vi "PicoScope6000aGetTriggerInfo.vi"(0 "handle in":i16, 5 "Segment Range":T1={"fromSegmentIndex"=0, "toSegmentIndex"=9} {"toSegmentIndex" format="%.4p"; "fromSegmentIndex" format="%.4p"}, 9 "Sample Rate":dbl, 11 "error in":errorcluster) -> (4 "handle out":i16, 6 "Trigger Info":T2(array[cluster]), 10 "Trigger Offsets":cluster{"Samples":u64, "Time (seconds)":dbl}[](array[cluster]) {"Time (seconds)" format="%#_5p"}, 15 "error out":errorcluster)   [LabVIEW 2010]
doc: "This VI gets a set of blocks captured using rapid block mode. It outputs two-dimensional arrays for each channel that contain data from all the requested captures."
uses:
  ps6000a.dll
  shared/Segment Range.ctl
panel:
  out "Number of Captures":u64=1
  out "fromSegmentIndex":u64
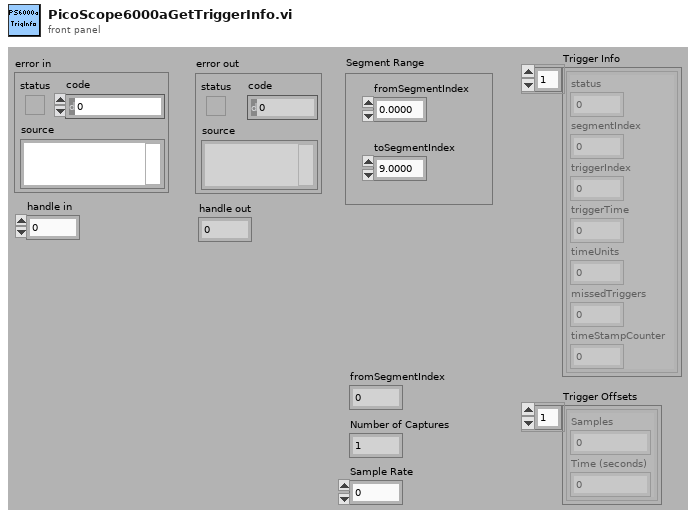
[diagram p1: front panel]
types:
  T1 = typedef "Segment Range.ctl" = cluster{"fromSegmentIndex":u64, "toSegmentIndex":u64}
  T2 = cluster{"status":u32, "segmentIndex":u64, "triggerIndex":u64, "triggerTime":dbl, "timeUnits":u32, "missedTriggers":u64, "timeStampCounter":u64}[]
  T3 = cluster{"status":u32, "segmentIndex":u64, "triggerIndex":u64, "triggerTime":dbl, "timeUnits":u32, "missedTriggers":u64, "timeStampCounter":u64}
  T4 = cluster{"status":bool, "code":u32, "source":string}
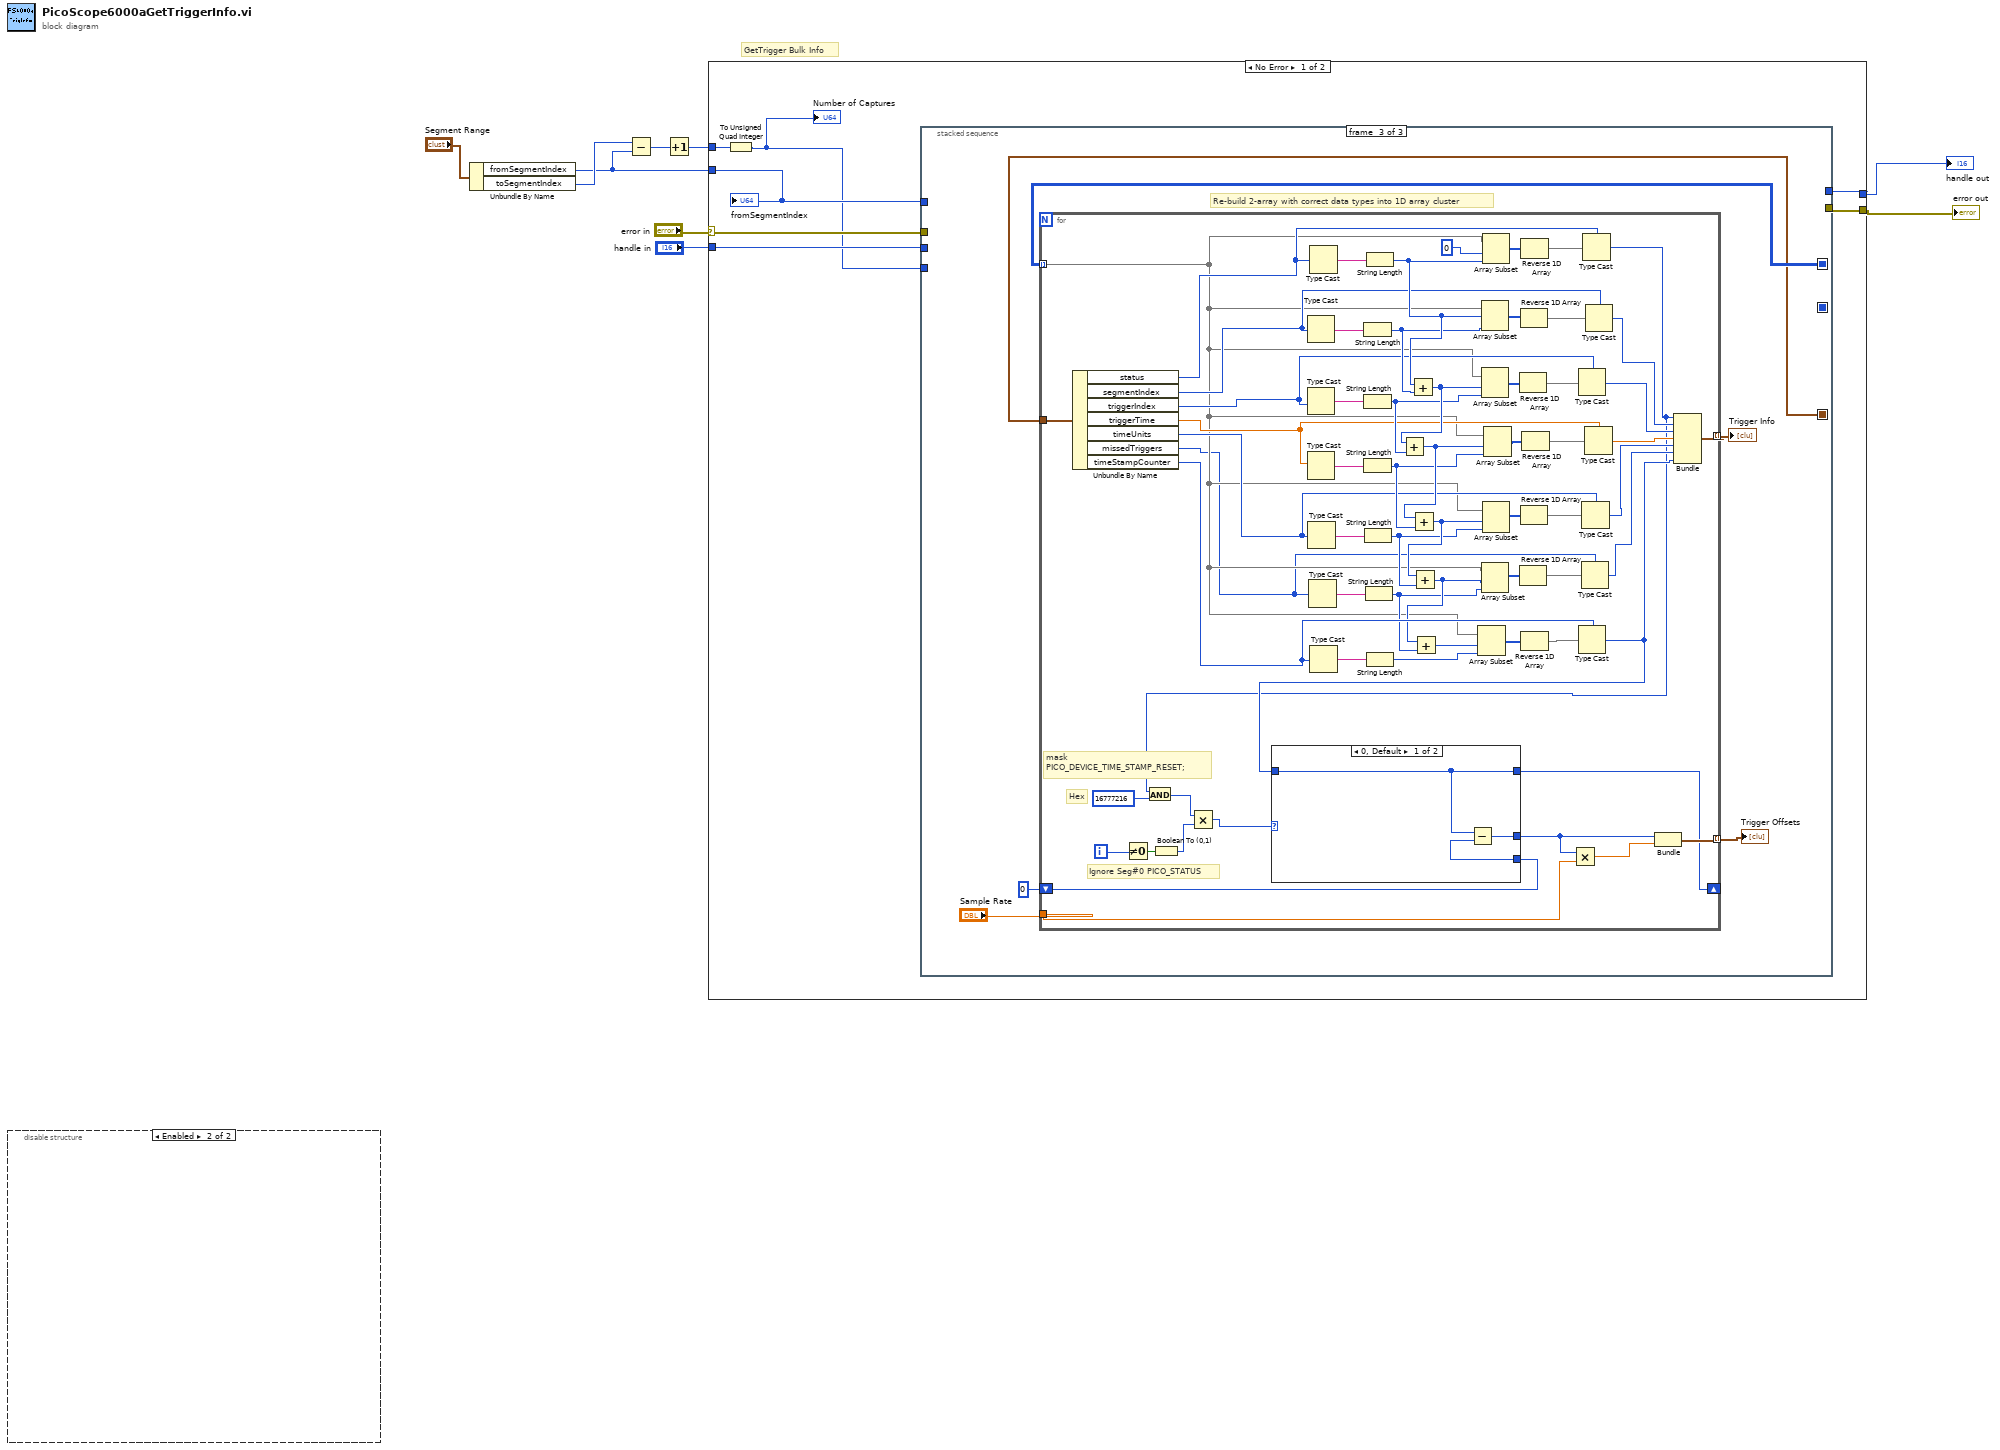
[diagram p0: block diagram]
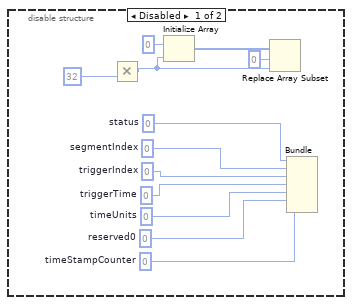
[diagram p2: hidden frame]
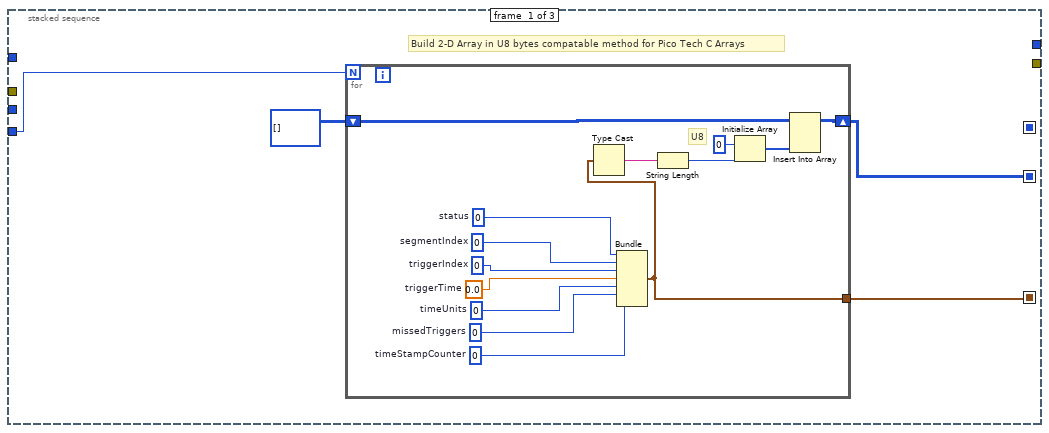
[diagram p3: hidden frame]
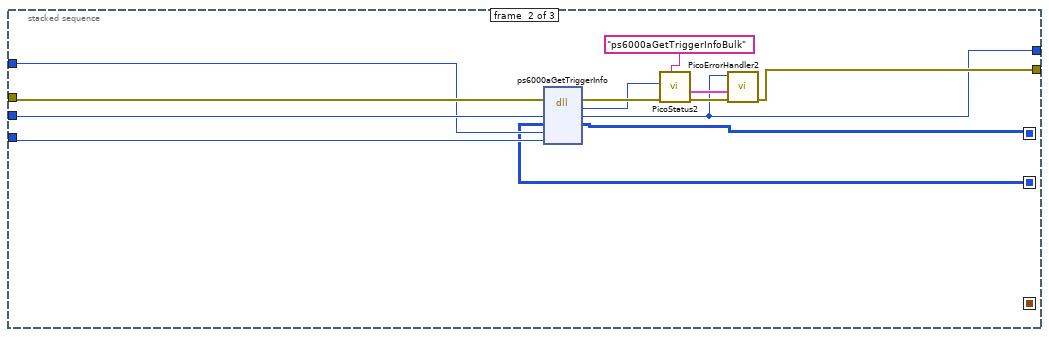
[diagram p4: hidden frame]
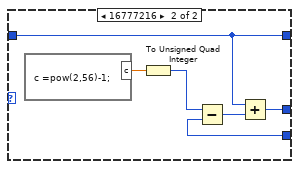
[diagram p5: hidden frame]
diagram:
  # "GetTrigger Bulk Info"
  n1 = disable-structure shown="Enabled" {
    frame Disabled {
      w17 = u64 0  # timeStampCounter
      w15 = i16 0  # reserved0
      w16 = i16 0  # timeUnits
      w18 = i64 0  # triggerTime
      w19 = u32 0  # triggerIndex
      w20 = u32 0  # segmentIndex
      w21 = u32 0  # status
      n2 = Multiply(y=u32 32) -> (x*y=w13:u32)  [unwired: 1 in]
      n3 = Initialize Array(u8 0 ("element"), w13) -> (w14:u8[])
      n4 = Replace Array Subset(array=w14, new element=w13, index=0) -> ()  [unwired: 1 out]
      n5 = Bundle("status"=w21, "segmentIndex"=w20, "triggerIndex"=w19, "triggerTime"=w18, "timeUnits"=w16, "reserved0"=w15, "timeStampCounter"=w17) -> ()  [unwired: 1 in, 1 out]
    }
    frame Enabled {
    }
  }
  n6 = Unbundle By Name("Segment Range") -> ("fromSegmentIndex"=w5:u64, "toSegmentIndex"=w6:u64)
  n7 = Subtract(x=w6, y=w5) -> (x-y=w4:u64)
  n8 = Increment(x=w4) -> (x+1=w3:u64)
  n9 = case shown="No Error" "error in" {
    selector: "error in" -> [w28 w140]
    tunnel: [w26 w140] -> w1
    tunnel: "handle in" -> [w27 w139]
    tunnel: [w25 w139] -> w7
    tunnel: w3 -> [w24 _]
    tunnel: w5 -> [w23 _]
    frame No Error {
      n10 = To Unsigned Quad Integer(1:w24) -> (0:w22:u64)
      "Number of Captures" <- w22
      n11 = stacked-sequence {
        seq-local: [w31 _ _] -> [_ w53 _]
        seq-local: [w30 _ _] -> [_ w51 _]
        seq-local: [_ w52 _] -> [_ _ w66]
        seq-local: [_ w51 _] -> [_ _ w63]
        tunnel: w28 -> [_ w57 _]
        tunnel: w27 -> [_ w56 _]
        tunnel: w23 -> [_ w55 _]
        tunnel: w22 -> [w29 w54 _]
        tunnel: [_ w48 _] -> w26
        tunnel: [_ w47 _] -> w25
        frame #0 {
          # "Build 2-D Array in U8 bytes compatable method for Pico Tech C Arrays"
          n12 = for {
            N: w29 -> [_]
            shift-right: [w34] -> w31
            shift-left: u8[][] [] -> [w35]
            tunnel: [w33] -> w30
            w42 = u64 0  # timeStampCounter
            w40 = u64 0  # missedTriggers
            w41 = u32 0  # timeUnits
            w43 = 0.0  # triggerTime
            w44 = u64 0  # triggerIndex
            w45 = u64 0  # segmentIndex
            w46 = u32 0  # status
            # "U8"
            n13 = Bundle("status"=w46, "segmentIndex"=w45, "triggerIndex"=w44, "triggerTime"=w43, "timeUnits"=w41, "missedTriggers"=w40, "timeStampCounter"=w42) -> (w33:T3)  [unwired: 1 in]
            n14 = Type Cast(x=w33) -> (*(type *) &x=w39:string)  [unwired: 1 in]
            n15 = String Length(string=w39) -> (length=w37:i32)
            n16 = Initialize Array(u8 0 ("element"), w37) -> (w36:u8[])
            n17 = Insert Into Array(array=w35, new element=w36) -> (w34:u8[][])  [unwired: 2 in]
          }
        }
        frame #1 {
          n18 = dll-call lib="ps6000a.dll" fn="ps6000aGetTriggerInfo" ("ps3000.dll:_ps3000_open_unit@0")(error in=w57, "handle"=w56, "triggerInfo"=w53, "firstSegmentIndex"=w55, "segmentCount"=w54) -> (error out=w60:errorcluster, "PICO_STATUS"=w59:u32, "handle"=w47:i16, "triggerInfo"=w52:u8[][])  [unwired: 4 in, 1 out]
          n19 = call "PicoStatus2.vi"("PICO source"="ps6000aGetTriggerInfoBulk" ("source"), "Error in"=w60, "PICO STATUS"=w59) -> ("error out"=w50:errorcluster, "PICO_STATUS out"=w49:T4)  [unwired: 5 in]
          n20 = call "PicoErrorHandler2.vi"("error in (no error)"=w50, "PICO_STATUS in"=w49, "handle In"=w47) -> ("error out"=w48:errorcluster)  [unwired: 8 in]
        }
        frame #2 {
          # "Re-build 2-array with correct data types into 1D array cluster"
          n21 = for {
            tunnel: w66 -> [w80] mode=indexing
            tunnel: [w126] -> w62 mode=indexing
            tunnel: [w113] -> w65 mode=indexing
            tunnel: "Sample Rate" -> [w112]
            tunnel: w63 -> [w91]
            shift-right: [w71] -> _
            shift-left: u64 0 ("timeStampCounter") -> [w72]
            i -> [w67]
            # "Hex"
            # "mask\nPICO_DEVICE_TIME_STAMP_RESET;"
            # "Ignore Seg#0 PICO_STATUS"
            n22 = Unbundle By Name(w91) -> ("status"=w90:u32, "segmentIndex"=w89:u64, "triggerIndex"=w85:u64, "triggerTime"=w86:dbl, "timeUnits"=w87:u32, "missedTriggers"=w79:u64, "timeStampCounter"=w88:u64)
            n23 = Not Equal To 0?(x=w67) -> (x != 0?=w77:bool)
            n24 = Boolean To (0,1)(Boolean=w77) -> (0, 1=w76:i16)
            n25 = Type Cast(x=w89) -> (*(type *) &x=w109:string)  [unwired: 1 in]
            n26 = Type Cast(x=w85) -> (*(type *) &x=w108:string)  [unwired: 1 in]
            n27 = Type Cast(x=w86) -> (*(type *) &x=w107:string)  [unwired: 1 in]
            n28 = Type Cast(x=w87) -> (*(type *) &x=w106:string)  [unwired: 1 in]
            n29 = Type Cast(x=w79) -> (*(type *) &x=w105:string)  [unwired: 1 in]
            n30 = Type Cast(x=w90) -> (*(type *) &x=w110:string)  [unwired: 1 in]
            n31 = Type Cast(x=w88) -> (*(type *) &x=w100:string)  [unwired: 1 in]
            n32 = String Length(string=w109) -> (length=w96:i32)
            n33 = String Length(string=w108) -> (length=w94:i32)
            n34 = String Length(string=w107) -> (length=w93:i32)
            n35 = String Length(string=w106) -> (length=w92:i32)
            n36 = String Length(string=w105) -> (length=w83:i32)
            n37 = String Length(string=w110) -> (length=w101:i32)
            n38 = String Length(string=w100) -> (length=w98:i32)
            n39 = Add(x=w101, y=w96) -> (x+y=w95:i32)
            n40 = Add(x=w95, y=w94) -> (x+y=w104:i32)
            n41 = Add(x=w104, y=w93) -> (x+y=w103:i32)
            n42 = Add(x=w103, y=w92) -> (x+y=w84:i32)
            n43 = Add(x=w84, y=w83) -> (x+y=w99:i32)
            n44 = Array Subset(array=w80, index=w99, length=w98) -> (w97:u8[])
            n45 = Array Subset(array=w80, index=w101, length=w96) -> (w125:u8[])
            n46 = Array Subset(array=w80, index=w95, length=w94) -> (w120:u8[])
            n47 = Array Subset(array=w80, index=w84, length=w83) -> (w81:u8[])
            n48 = Array Subset(array=w80, index=0, length=w101) -> (w123:u8[])
            n49 = Array Subset(array=w80, index=w103, length=w92) -> (w117:u8[])
            n50 = Array Subset(array=w80, index=w104, length=w93) -> (w119:u8[])
            n51 = Reverse 1D Array(array=w120) -> (reversed array=w121:u8[])
            n52 = Reverse 1D Array(array=w81) -> (reversed array=w82:u8[])
            n53 = Reverse 1D Array(array=w125) -> (reversed array=w124:u8[])
            n54 = Reverse 1D Array(array=w117) -> (reversed array=w116:u8[])
            n55 = Reverse 1D Array(array=w123) -> (reversed array=w122:u8[])
            n56 = Reverse 1D Array(array=w97) -> (reversed array=w115:u8[])
            n57 = Reverse 1D Array(array=w119) -> (reversed array=w118:u8[])
            n58 = Type Cast(type=w85, x=w121) -> (*(type *) &x=w129:u64)
            n59 = Type Cast(type=w88, x=w115) -> (*(type *) &x=w70:u64)
            n60 = Type Cast(type=w79, x=w82) -> (*(type *) &x=w78:u64)
            n61 = Type Cast(type=w87, x=w116) -> (*(type *) &x=w127:u32)
            n62 = Type Cast(type=w90, x=w122) -> (*(type *) &x=w69:u32)
            n63 = And(x=w69, y=u32 16777216) -> (x .and. y?=w75:u32)
            n64 = Multiply(x=w75, y=w76) -> (x*y=w68:u32)
            n65 = case shown="0, Default" w68 {
              tunnel: w70 -> [w131 w136]
              tunnel: [w131 w136] -> w71
              tunnel: w72 -> [w130 w138]
              tunnel: [w132 w135] -> w73
              frame 0, Default {
                n66 = Subtract(x=w131, y=w130) -> (x-y=w132:u64)
              }
              frame 16777216 {
                n67 = formula code="c =pow(2,56)-1;"() -> ("c"=w134:dbl)
                n68 = To Unsigned Quad Integer(1:w134) -> (0:w133:u64)
                n69 = Subtract(x=w133, y=w138) -> (x-y=w137:u64)
                n70 = Add(x=w136, y=w137) -> (x+y=w135:u64)
              }
            }
            n71 = Multiply(x=w73, y=w112) -> (x*y=w111:dbl)
            n72 = Type Cast(type=w86, x=w118) -> (*(type *) &x=w128:dbl)
            n73 = Type Cast(type=w89, x=w124) -> (*(type *) &x=w114:u64)
            n74 = Bundle(w73, w111) -> (w113:cluster{u64, dbl})  [unwired: 1 in]
            n75 = Bundle("status"=w69, "segmentIndex"=w114, "triggerIndex"=w129, "triggerTime"=w128, "timeUnits"=w127, "missedTriggers"=w78, "timeStampCounter"=w70) -> (w126:T3)  [unwired: 1 in]
          }
          "Trigger Offsets" <- w65
          "Trigger Info" <- w62
        }
      }
      "fromSegmentIndex" <- w23
    }
    frame Error {
    }
  }
  "handle out" <- w7
  "error out" <- w1
